vi "RVC Drive in Circles Maneuver.vi"() -> ()   [LabVIEW 2017]
uses:
  <vilib>/Simulation/Scripting/Companion Diagram/SimConfigNode/SimParams.ctl
  <vilib>/Simulation/Scripting/Companion Diagram/SimConfigNode/_simSolvers.ctl
  <vilib>/Simulation/Implementation/Shared/SIMSCR Execution Mode.ctl
  <vilib>/Simulation/Param Hierarchy/Typedefs/SIMPH Param Control Actions.ctl
  <vilib>/Simulation/Scripting/Editor Utilities/SIM subVI tag data.ctl
  <vilib>/Simulation/Scripting/Editor Utilities/SIM subVI execution type.ctl
  <vilib>/Simulation/Implementation/Shared/NILVSim_ParamChanged.vi
  <vilib>/Simulation/Implementation/Shared/NILVSIM_BeginStep.vi
  <vilib>/Simulation/Utility/Implementation/SIM Time.vi
  <vilib>/Simulation/SignalArithmetic/Implementation/NILVSim Gain.llb/SIM Gain (scalar).vi
  <vilib>/Simulation/Utility/Implementation/NILVSim Collector.llb/SIM Collector (vector).vi
  <vilib>/Simulation/Utility/Implementation/NILVSim Collector.llb/SIM Collector (scalar).vi
  <vilib>/Analysis/coordinate.llb/Wrap Angle.vi
  <vilib>/Analysis/coordinate.llb/Wrap Angle (scalar).vi
  <vilib>/Simulation/Implementation/Shared/SIM Fire Discrete SubVI.vi
  <vilib>/Simulation/Implementation/Shared/NILVSim_Manager.vi
  <vilib>/Utility/error.llb/Clear Errors.vi
  <vilib>/Simulation/Implementation/Shared/NILVSim_FinalizeModel.vi
  <vilib>/Simulation/Utility/Implementation/NILVSim Collector.llb/NILVSim Collector core (vector).vi
  <vilib>/Simulation/Utility/Implementation/NILVSim Collector.llb/NILVSim Collector core (scalar).vi
  <vilib>/Simulation/Implementation/Shared/SIM Fire Discrete SubVI (Core).vi
  <vilib>/Simulation/Implementation/Shared/SIM Unbundle Sim Info.vi
  <vilib>/Simulation/Implementation/Shared/NILVSim_Initialize.vi
  <vilib>/Simulation/Utility/Implementation/NILVSim Get Time and IsAcceptedStep.vi
  <vilib>/addons/control/pid/pid.llb/PID Output Rate Limiter.vi
  <vilib>/addons/control/pid/pid.llb/PID Output Rate Limiter (DBL).vi
  penguin/lvaddon/robotics/branches/untargeted/Bordeaux/Book/Chapter 4/subVIs/2D Animate Rotating Wheel.vi
  penguin/lvaddon/robotics/branches/untargeted/Bordeaux/Book/Chapter 4/subVIs/2D Animation Plot.vi
  <vilib>/Simulation/Implementation/Shared/SIMSH Read Queue.vi
  <vilib>/Simulation/Implementation/Shared/NILVSim_GetModelError.vi
  <vilib>/Simulation/Implementation/Shared/SIM Bundle Sim Info.vi
  <vilib>/Simulation/Scripting/Companion Diagram/SimConfigNode/SimDog.xnode
  penguin/lvaddon/robotics/branches/untargeted/Bordeaux/Book/Chapter 4/SIM Bicycle.vi
  <vilib>/Simulation/Model Libraries/PID/SIM PID (Parallel).vi
  <vilib>/Simulation/Model Libraries/PID/SIM PID.vi
  <vilib>/Simulation/Implementation/XNodeFramework/SimXNode/SimX.xnode
  <vilib>/Analysis/NI_AAL_Angle.lvlib
  <vilib>/addons/control/pid/NI_PID_pid.lvlib
  <vilib>/Simulation/Implementation/Shared/NI_SIM_Implementation.lvlib
panel:
  in  "output rate (EGU/min)":dbl=33.0 format="%.2f"
  out "Steering":cluster{"Time":dbl[], "Signal":dbl[]}(graph)
  in  "target radius":dbl=2.0 format="%#_13g"
  in  "target speed":dbl=0.1 format="%#_13g"
  out "Coordinate Frame":cluster{dbl[], dbl[]}[](graph)
  out "Speed":cluster{"Time":dbl[], "Signal":dbl[]}(graph)
  out "Position":cluster{"Signal":dbl[], "Signal":dbl[]}(graph)
  out "Position":cluster{"x":dbl, "y":dbl, "theta":dbl}
  out "Angle (deg)":dbl format="%.2f"
  out "Steering Angle":picture
  out "Goal":dbl[](array[numeric])
  out "velocity":dbl(knob)=1.0 scale=0.0..10.0
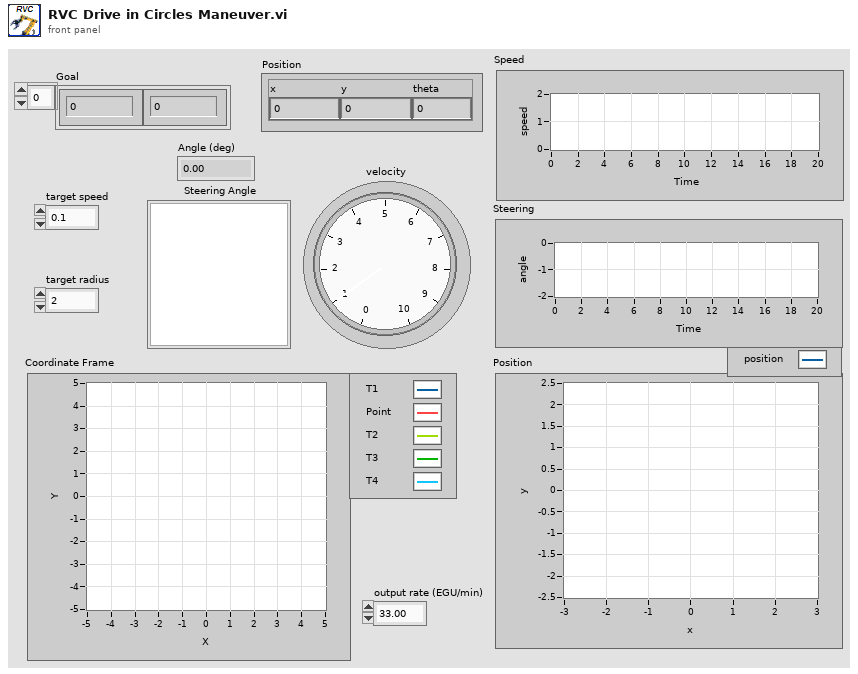
[diagram p1: front panel]
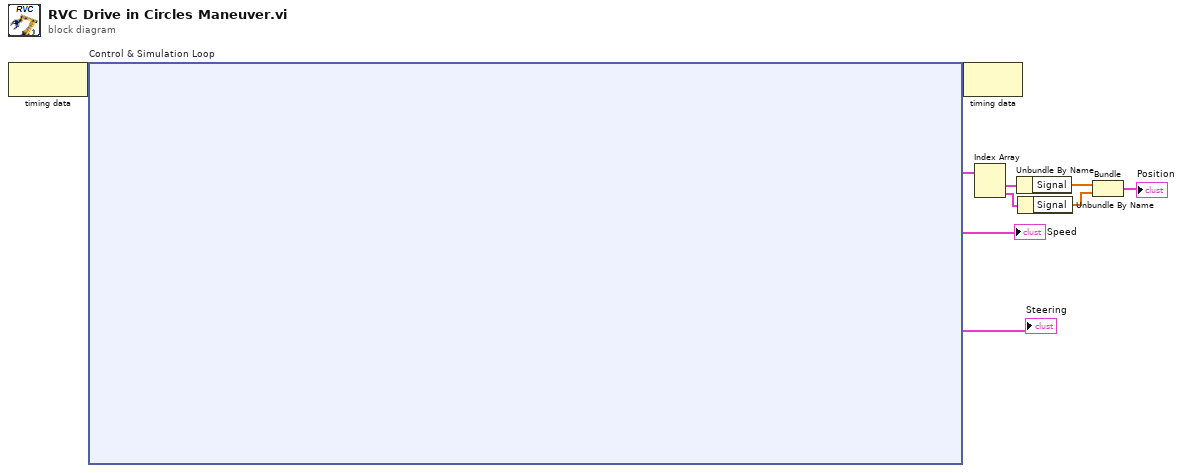
[diagram p0: block diagram]
diagram:
  n1 = node-c288() -> (w9:variant)  [unwired: 1 in]
  n2 = node-c254 "Control & Simulation Loop"(w9) -> (w8:variant, w7:cluster{"Time":dbl[], "Signal":dbl[]}[], →"Speed":cluster{"Time":dbl[], "Signal":dbl[]}, →"Steering":cluster{"Time":dbl[], "Signal":dbl[]})
  n3 = node-c288(w8) -> ()  [unwired: 1 out]
  n4 = Index Array(array=w7) -> (element #1=w6:cluster{"Time":dbl[], "Signal":dbl[]}, element #2=w5:cluster{"Time":dbl[], "Signal":dbl[]})  [unwired: 2 in]
  n5 = Unbundle By Name(w6) -> ("Signal"=w4:dbl[])
  n6 = Unbundle By Name(w5) -> ("Signal"=w3:dbl[])
  n7 = Bundle("Signal"=w4, "Signal"=w3) -> (→"Position":cluster{"Signal":dbl[], "Signal":dbl[]})  [unwired: 1 in]
